vi "CALCULO_CHECKSUM.vi"() -> ()   [LabVIEW 2018]
panel:
  out "DATOS":string
  out "DEC":u32
  out "x .xor. y?":u32
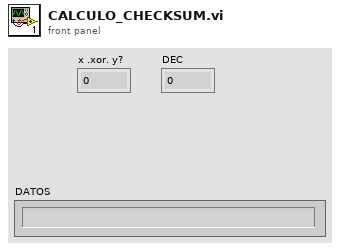
[diagram p1: front panel]
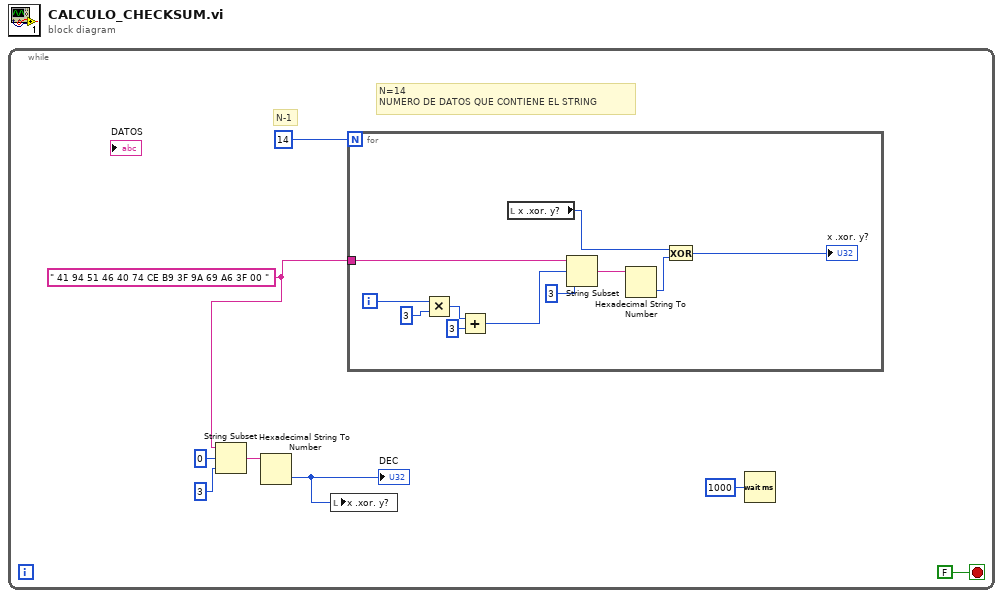
[diagram p0: block diagram]
diagram:
  n1 = while {
    stop <- FALSE stop-if-true
    w1 = " 41 94 51 46 40 74 CE B9 3F 9A 69 A6 3F 00 " ("DATOS")
    # "N-1"
    # "N=14 \nNUMERO DE DATOS QUE CONTIENE EL STRING"
    n2 = String Subset(string=w1, offset (0)=0, length (rest)=3 ("length (rest)")) -> (substring=w4:string)
    n3 = Hexadecimal String To Number(string=w4) -> (number=w7:u32)  [unwired: 2 in, 1 out]
    "DEC" <- w7
    n4 = local write "x .xor. y?"(w7) -> ()
    n5 = for {
      N: 14 -> [_]
      tunnel: w1 -> [w9]
      i -> [w14]
      n6 = Multiply(x=w14, y=3) -> (x*y=w12:i32)
      n7 = Add(x=w12, y=3) -> (x+y=w11:i32)
      n8 = local read "x .xor. y?"() -> (w17:u32)
      n9 = String Subset(string=w9, offset (0)=w11, length (rest)=3 ("length (rest)")) -> (substring=w18:string)
      n10 = Hexadecimal String To Number(string=w18) -> (number=w16:u32)  [unwired: 2 in, 1 out]
      n11 = Exclusive Or(1:w16, 2:w17) -> (0:→"x .xor. y?":u32)
    }
    n12 = Wait (ms)(milliseconds to wait=u32 1000) -> ()  [unwired: 1 out]
  }
